vi "Write Auto Grow.vi"(8 "error in (no error)":errorcluster, 10 "Auto Grow?":bool, 11 "TabControl.lvclass in":refnum<class "TabControl.lvclass">) -> (0 "error out":errorcluster, 3 "TabControl.lvclass out":refnum<class "TabControl.lvclass">)   [LabVIEW 2015, in "TabControl.lvclass"]
uses:
  TabControl.lvclass
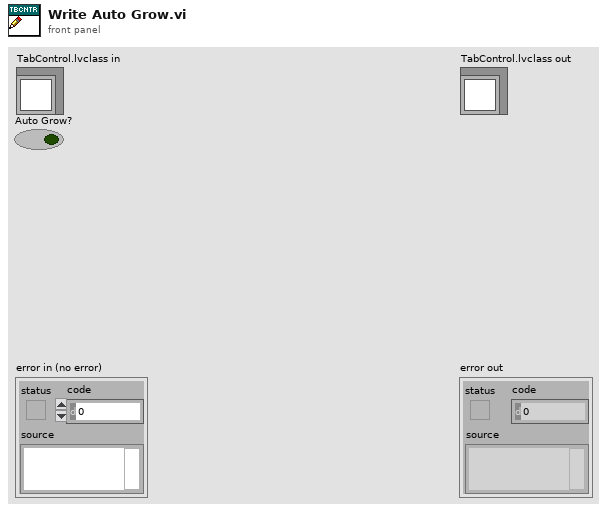
[diagram p1: front panel]
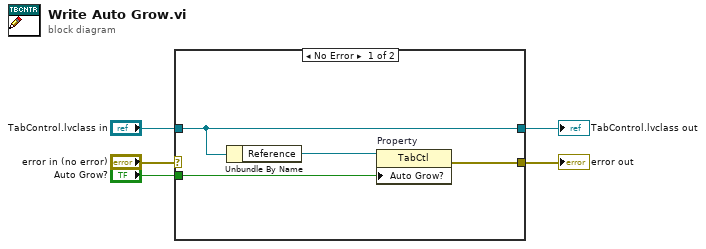
[diagram p0: block diagram]
diagram:
  n1 = case shown="No Error" "error in (no error)" {
    selector: "error in (no error)" -> [_ w11]
    tunnel: [w9 w11] -> w4
    tunnel: [w7 w10] -> w2
    tunnel: "TabControl.lvclass in" -> [w7 w10]
    tunnel: "Auto Grow?" -> [w8 _]
    frame No Error {
      n2 = Unbundle By Name(w7) -> ("Reference"=w6:refnum<vi>)
      n3 = property on="Property" class="TabCtl"(reference=w6, "Auto Grow?"=w8) -> (error out=w9:errorcluster)  [unwired: 1 in, 1 out]
    }
    frame Error {
    }
  }
  "error out" <- w4
  "TabControl.lvclass out" <- w2
